vi "testEXT Failes If Element Is Not Found At Given Index.vi"(8 "error in (no error)":errorcluster, 11 "TestCase in":refnum<class "Search In 1D Array Test Case.lvclass">) -> (0 "error out":errorcluster, 3 "TestCase out":refnum<class "Search In 1D Array Test Case.lvclass">)   [LabVIEW 2015, in "Search In 1D Array Test Case.lvclass"]
uses:
  Search In 1D Array Test Case.lvclass
  SubVIs/Search in array/Pass If In 1D Array (EXT).vi
  <vilib>/addons/_JKI Toolkits/VI Tester/TestCase.llb/TestCase.lvclass
  VITAC.lvlib
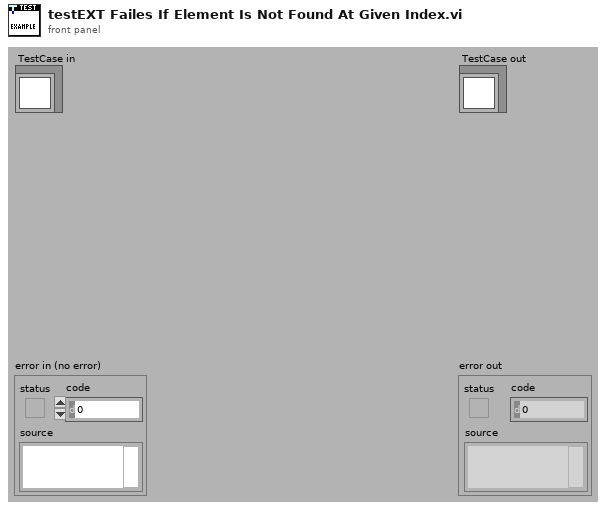
[diagram p1: front panel]
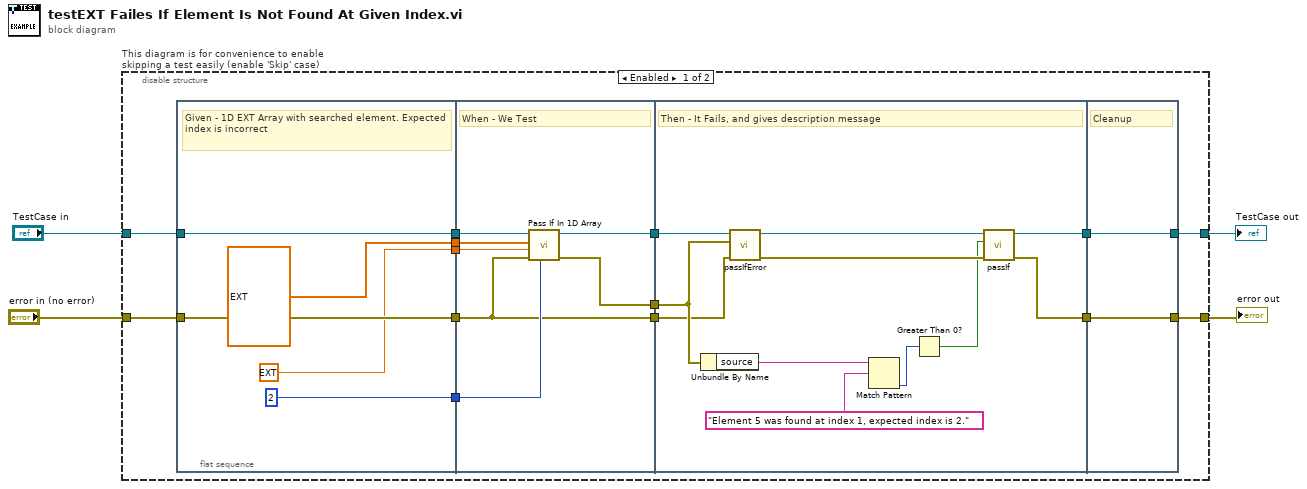
[diagram p0: block diagram]
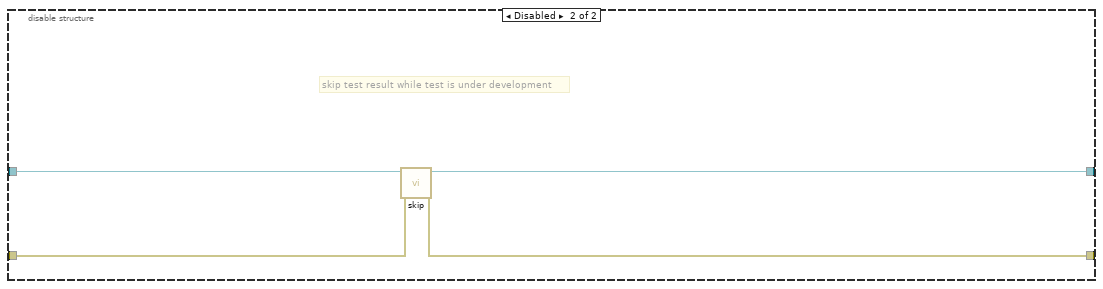
[diagram p2: hidden frame]
diagram:
  n1 = disable-structure "This diagram is for convenience to enable skipping a test easily (enable 'Skip' case)" shown="Enabled" {
    disable-tunnel: "TestCase in" -> [w10 w47]
    disable-tunnel: [w13 w45] -> w1
    disable-tunnel: [w12 w46] -> w3
    disable-tunnel: "error in (no error)" -> [w11 w44]
    frame Enabled {
      n2 = flat-sequence {
        tunnel: w11 -> [w22]
        tunnel: w10 -> [w23]
        tunnel: [w23] -> w18
        tunnel: [w22] -> w17
        tunnel: [ext 5.0] -> w9
        tunnel: [ext[] [1.0, 5.0, 10.0, 20.5]] -> w8
        tunnel: [2] -> w7
        tunnel: [w29] -> w16
        tunnel: [w28] -> w15
        tunnel: w18 -> [w30]
        tunnel: w17 -> [w24]
        tunnel: w9 -> [w27]
        tunnel: w8 -> [w26]
        tunnel: w7 -> [w25]
        tunnel: [w24] -> w6
        tunnel: [w32] -> w14
        tunnel: w16 -> [w35]
        tunnel: w15 -> [w34]
        tunnel: w6 -> [w33]
        tunnel: [w31] -> w5
        tunnel: [w42] -> w12
        tunnel: [w43] -> w13
        tunnel: w14 -> [w43]
        tunnel: w5 -> [w42]
        frame #0 {
          # "Given - 1D EXT Array with searched element. Expected index is incorrect"
        }
        frame #1 {
          # "When - We Test"
          n3 = call-poly "Pass If In 1D Array.vi"("expected index (optional)"=w25, "error in (no error)"=w24, "element"=w27, "1D array"=w26, "TestCase in"=w30) -> ("error out"=w28:errorcluster, "TestCase out"=w29:refnum<class "Search In 1D Array Test Case.lvclass">)  [unwired: 5 in]
        }
        frame #2 {
          # "Then - It Fails, and gives description message"
          n4 = Unbundle By Name(w34) -> ("source"=w39:string)
          n5 = call-dynamic "passIfError.vi"("error in (no error)"=w33, "error"=w34, "TestCase in"=w35) -> ("error out"=w40:errorcluster, "TestCase out"=w41:refnum<class "Search In 1D Array Test Case.lvclass">)  [unwired: 7 in]
          n6 = Match Pattern(string=w39, regular expression="Element 5 was found at index 1, expected index is 2.") -> (offset past match=w37:i32)  [unwired: 1 in, 3 out]
          n7 = Greater Than 0?(x=w37) -> (x > 0?=w36:bool)
          n8 = call-dynamic "passIf.vi"("error in (no error)"=w40, "pass"=w36, "TestCase in"=w41) -> ("error out"=w31:errorcluster, "TestCase out"=w32:refnum<class "Search In 1D Array Test Case.lvclass">)  [unwired: 7 in]
        }
        frame #3 {
          # "Cleanup"
        }
      }
    }
    frame Disabled {
      # "skip test result while test is under development"
      n9 = call <vilib>:"skip.vi"("error in (no error)"=w44, "TestCase in"=w47) -> ("error out"=w46:errorcluster, "TestCase out"=w45:refnum<class "Search In 1D Array Test Case.lvclass">)  [unwired: 8 in]
    }
  }
  "error out" <- w3
  "TestCase out" <- w1
